vi "Do.vi"(8 "error in (no error)":errorcluster, 10 "Actor in":refnum<class "Actor.lvclass">, 11 "Register Actor":refnum<class "Register Actor Msg.lvclass">) -> (0 "error out":errorcluster, 2 "Actor out":refnum<class "Actor.lvclass">)   [LabVIEW 2020, in "AF Debug.lvlib" / "Register Actor Msg.lvclass"]
doc: "This VI delivers the Registration message to the actor. Unlike most messages, it does NOT invoke a method on the actor class."
uses:
  Register Actor Msg.lvclass
  vi.lib/ActorFramework/Actor/Actor.lvclass
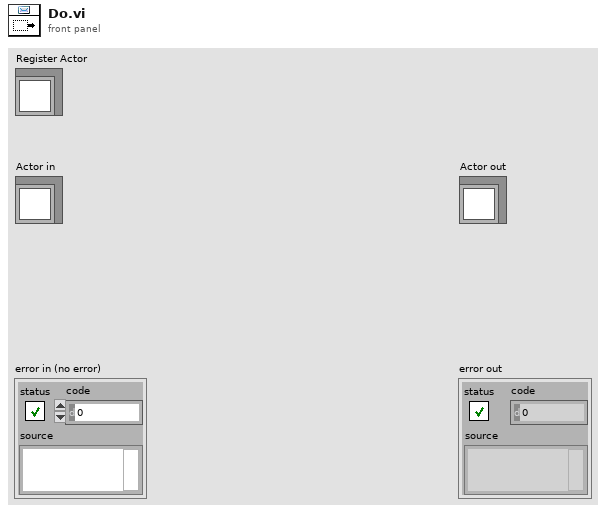
[diagram p1: front panel]
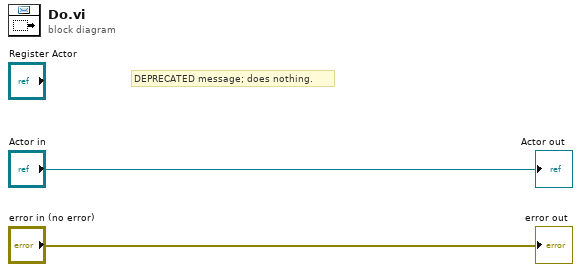
[diagram p0: block diagram]
diagram:
  # "DEPRECATED message; does nothing."
  "error out" <- "error in (no error)"
  "Actor out" <- "Actor in"
